vi "WfmDataAccessor SearchIndex.vi"(8 "error in (no error)":errorcluster, 9 "XML in":string, 11 "WfmDataAccessor in":refnum<class "WfmDataAccessor.lvclass">) -> (0 "error out":errorcluster, 1 "filename":string, 2 "Found":bool, 3 "WfmDataAccessor out":refnum<class "WfmDataAccessor.lvclass">)   [LabVIEW 2018, in "WfmDataAccessor.lvclass"]
uses:
  WfmDataAccessor.lvclass
  WfmDataAccessor.lvclass/WfmDataAccessor.ctl
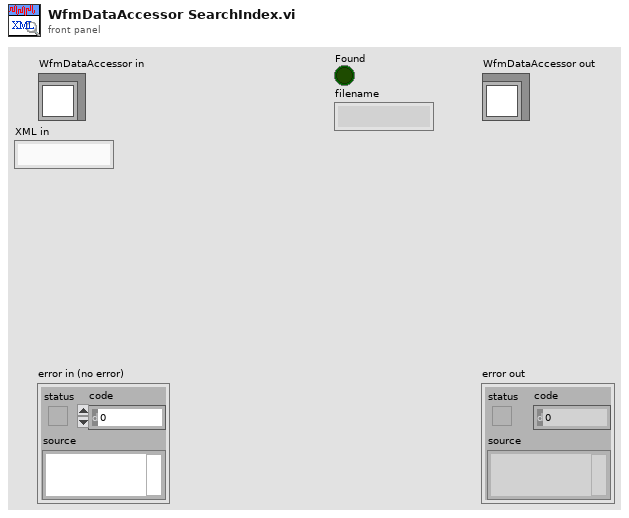
[diagram p1: front panel]
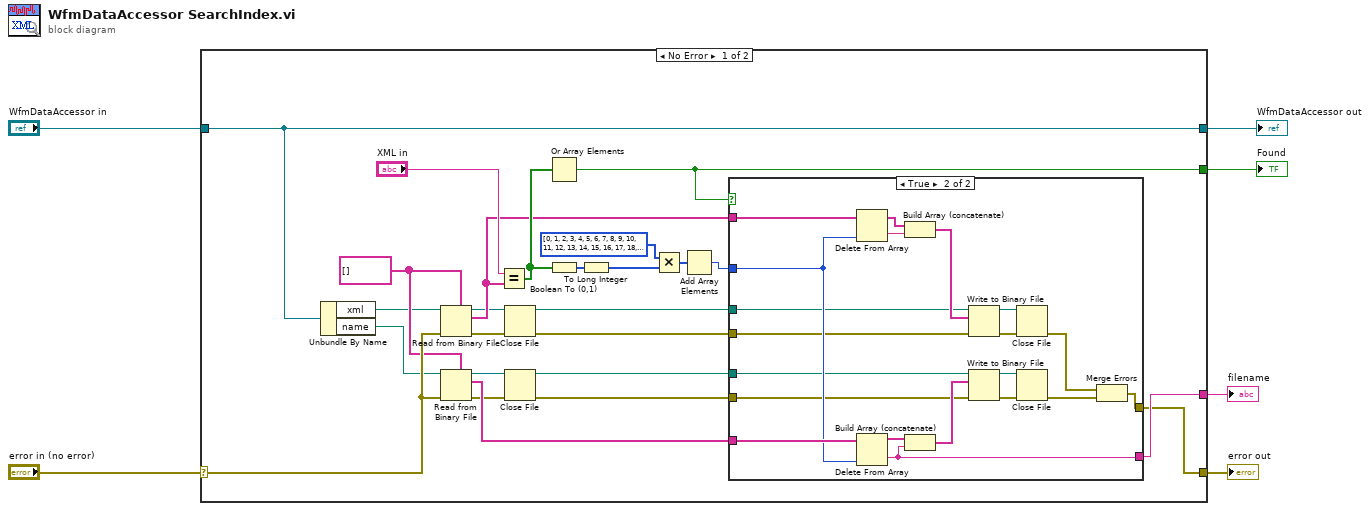
[diagram p0: block diagram]
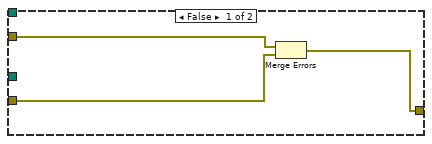
[diagram p2: hidden frame]
diagram:
  n1 = case shown="No Error" "error in (no error)" {
    selector: "error in (no error)" -> [w22 w56]
    tunnel: [w7 w56] -> w5
    tunnel: [w31 w55] -> w3
    tunnel: "WfmDataAccessor in" -> [w31 w55]
    tunnel: [w24 _] -> w2
    tunnel: [w18 _] -> w1
    frame No Error {
      w21 = string[] [] ("XML")
      n2 = Unbundle By Name(w31) -> ("xml"=w17:path, "name"=w16:path)
      n3 = Read from Binary File(5:w21, 8:w22, 11:w17) -> (0:w14:errorcluster, 2:w20:string[], 3:w15:refnum<file>)  [unwired: 3 in, 1 out]
      n4 = Read from Binary File(5:w21, 8:w22, 11:w16) -> (0:w12:errorcluster, 2:w19:string[], 3:w13:refnum<file>)  [unwired: 3 in, 1 out]
      n5 = Equal?(x="XML in", y=w20) -> (x = y?=w25:bool[])
      n6 = Close File(refnum=w15, error in=w14) -> (path=w11:path, error out=w8:errorcluster)
      n7 = Close File(refnum=w13, error in=w12) -> (path=w10:path, error out=w9:errorcluster)
      n8 = Or Array Elements(Boolean array=w25) -> (logical OR=w24:bool)
      n9 = Boolean To (0,1)(Boolean=w25) -> (0, 1=w29:i16[])
      n10 = To Long Integer(number=w29) -> (32bit integer=w27:i32[])
      n11 = Multiply(x=i32[] [0, 1, 2, 3, 4, 5, 6, 7, 8, 9, 10, 11, 12, 13, 14, 15, 16, 17, 18, 19, 20, 21, 22, 23, 24, 25, 26, 27, 28, 29, 30, 31, 32, 33, 34, 35, 36, 37, 38, 39, 40, 41, 42, 43, 44, 45, 46, 47, 48, 49, 50, 51, 52, 53, 54, 55, 56, 57, 58, 59, 60, 61, 62, 63, 64, 65, 66, 67, 68, 69, 70, 71, 72, 73, 74, 75, 76, 77, 78, 79, 80, 81, 82, 83, 84, 85, 86, 87, 88, 89, 90, 91, 92, 93, 94, 95, 96, 97, 98, 99, 100, 101, 102, 103, 104, 105, 106, 107, 108, 109, 110, 111, 112, 113, 114, 115, 116, 117, 118, 119, 120, 121, 122, 123, 124, 125, 126, 127, 128, 129, 130, 131, 132, 133, 134, 135, 136, 137, 138, 139, 140, 141, 142, 143, 144, 145, 146, 147, 148, 149, 150, 151, 152, 153, 154, 155, 156, 157, 158, 159, 160, 161, 162, 163, 164, 165, 166, 167, 168, 169, 170, 171, 172, 173, 174, 175, 176, 177, 178, 179, 180, 181, 182, 183, 184, 185, 186, 187, 188, 189, 190, 191, 192, 193, 194, 195, 196, 197, 198, 199] ("Array"), y=w27) -> (x*y=w26:i32[])
      n12 = Add Array Elements(numeric array=w26) -> (sum=w23:i32)
      n13 = case shown="True" w24 {
        tunnel: w23 -> [_ w52]
        tunnel: w20 -> [_ w54]
        tunnel: w19 -> [_ w53]
        tunnel: w11 -> [_ w49]
        tunnel: [_ w35] -> w18
        tunnel: w10 -> [_ w46]
        tunnel: w9 -> [w33 w45]
        tunnel: w8 -> [w34 w44]
        tunnel: [w32 w39] -> w7
        frame False {
          n14 = Merge Errors(w34, w33) -> (w32:errorcluster)
        }
        frame True {
          n15 = Delete From Array(array=w54, index=w52) -> (deleted portion=w37:string, array with subset deleted=w38:string[])  [unwired: 1 in]
          n16 = Delete From Array(array=w53, index=w52) -> (deleted portion=w35:string, array with subset deleted=w36:string[])  [unwired: 1 in]
          n17 = Build Array (concatenate)(w38, w37) -> (w50:string[])
          n18 = Build Array (concatenate)(w36, w35) -> (w51:string[])
          n19 = Write to Binary File(file (use dialog)=w49, data=w50, error in=w44) -> (refnum out=w48:refnum<file>, error out=w47:errorcluster)  [unwired: 3 in, 1 out]
          n20 = Write to Binary File(file (use dialog)=w46, data=w51, error in=w45) -> (refnum out=w43:refnum<file>, error out=w42:errorcluster)  [unwired: 3 in, 1 out]
          n21 = Close File(refnum=w48, error in=w47) -> (error out=w41:errorcluster)  [unwired: 1 out]
          n22 = Close File(refnum=w43, error in=w42) -> (error out=w40:errorcluster)  [unwired: 1 out]
          n23 = Merge Errors(w41, w40) -> (w39:errorcluster)
        }
      }
    }
    frame Error {
    }
  }
  "error out" <- w5
  "WfmDataAccessor out" <- w3
  "Found" <- w2
  "filename" <- w1
